vi "Move Label.vi"(0 "FSM.Edge In":refnum<class "FSM.Edge.lvclass">, 7 "pointIndex":i32) -> (4 "FSM.Edge Out":refnum<class "FSM.Edge.lvclass">)   [LabVIEW 2020, in "FSM.Edge.lvclass"]
uses:
  FSM.Edge.lvclass
  FSM.Edge.lvclass/FSM.Edge.ctl
  FSM.Label/FSM.Label.lvclass/FSM.Label.ctl
  FSM.Label/Write Location.vi
  FSM.Label/FSM.Label.lvclass
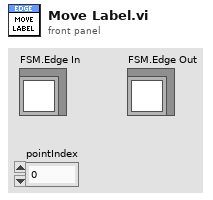
[diagram p1: front panel]
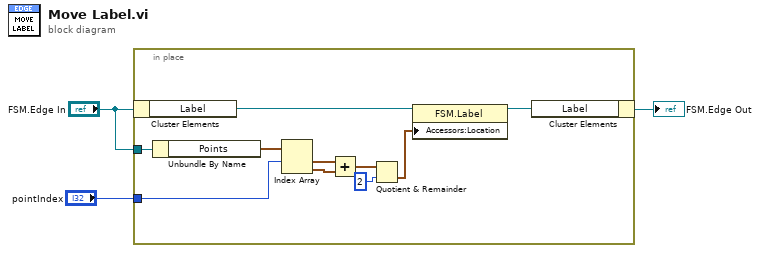
[diagram p0: block diagram]
diagram:
  n1 = in-place {
    in-place-border: "FSM.Edge In" -> [w11]
    in-place-border: "pointIndex" -> [w9]
    n2 = in-place-cluster #1("FSM.Edge In") -> ("Label"=w6:refnum<class "FSM.Label.lvclass">)
    n3 = Unbundle By Name(w11) -> ("Points"=w10:cluster{"x":i16, "y":i16}[])
    n4 = Index Array(array=w10, index #1=w9) -> (element #1=w8:cluster{"x":i16, "y":i16}, element #2=w7:cluster{"x":i16, "y":i16})  [unwired: 1 in]
    n5 = Add(x=w8, y=w7) -> (x+y=w13:cluster{"x":i16, "y":i16})
    n6 = Quotient & Remainder(x=w13, y=2) -> (floor(x/y)=w5:cluster{"x":i32, "y":i32})  [unwired: 1 out]
    n7 = property class="FSM.Label"(reference=w6, "Accessors:Location"=w5) -> (reference out=w4:refnum<class "FSM.Label.lvclass">)  [unwired: 1 in, 1 out]
    n8 = in-place-cluster #1("Label"=w4) -> (→"FSM.Edge Out":refnum<class "FSM.Edge.lvclass">)
  }
